vi "DigitalOut_read.vi"(8 "error in (no error)":errorcluster, 11 "DigitalOut in":refnum<class "DigitalOut.lvclass">) -> (0 "error out":errorcluster, 2 "value":bool, 3 "DigitalOut out":refnum<class "DigitalOut.lvclass">)   [LabVIEW 2011, in "mbed_LVLibrary.lvlib" / "DigitalOut.lvclass"]
uses:
  DigitalOut.lvclass
  DigitalOut.lvclass/DigitalOut.ctl
  Transport Mechanisms/mbed/mbed.lvclass
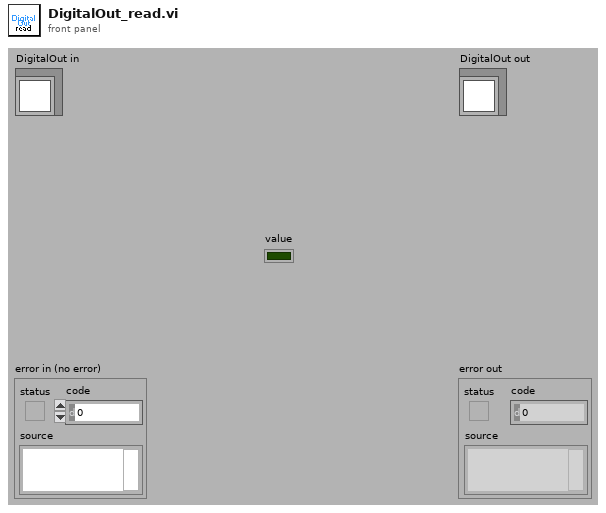
[diagram p1: front panel]
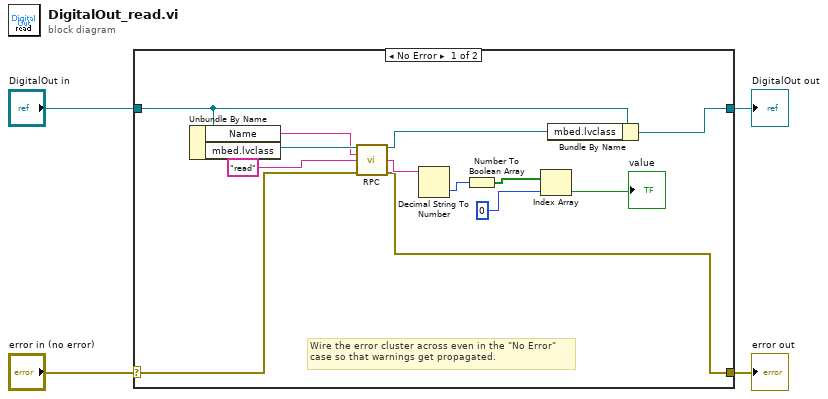
[diagram p0: block diagram]
diagram:
  n1 = case shown="No Error" "error in (no error)" {
    selector: "error in (no error)" -> [w6 w19]
    tunnel: [w5 w19] -> w3
    tunnel: [w16 w18] -> w1
    tunnel: "DigitalOut in" -> [w17 w18]
    frame No Error {
      # "Wire the error cluster across even in the \"No Error\"\ncase so that warnings get propagated."
      n2 = Unbundle By Name(w17) -> ("Name"=w14:string, "mbed.lvclass"=w15:refnum<class "mbed.lvclass">)
      n3 = call-dynamic "RPC.vi"("mbed in"=w15, "Name"=w14, "method"="read", "error in (no error)"=w6) -> ("mbed out"=w13:refnum<class "mbed.lvclass">, "RPC Result"=w9:string, "error out"=w5:errorcluster)  [unwired: 9 in]
      n4 = Decimal String To Number(string=w9) -> (number=w7:i32)  [unwired: 2 in, 1 out]
      n5 = Number To Boolean Array(number=w7) -> (Boolean array=w10:bool[])
      n6 = Index Array(array=w10, index=0) -> (element=→"value":bool)
      n7 = Bundle By Name(cluster=w17, "mbed.lvclass"=w13) -> (w16:refnum<class "DigitalOut.lvclass">)
    }
    frame Error {
    }
  }
  "error out" <- w3
  "DigitalOut out" <- w1
